vi "Read Coils.vi"(8 "error in (no error)":errorcluster, 9 "number of coils":u16, 10 "starting address":u16, 11 "Modbus master in":refnum<class "Modbus Master.lvclass">) -> (0 "error out":errorcluster, 2 "coil values":bool[](array[boolean]), 3 "Modbus master out":refnum<class "Modbus Master.lvclass">)   [LabVIEW 2020, in "Modbus Master.lvclass"]
doc: "Reads values from contiguous coils. The maximum number of coils this VI can read is 2,000."
uses:
  <vilib>/Modbus/master/Modbus Master.lvclass
  C:/builds/penguin/iak/lvdsc/trunk/20.0/lv/vi.lib/Modbus/subvis/Modbus API/Modbus API.lvclass
  <vilib>/Modbus/subvis/Modbus API/Modbus API.lvclass/Modbus API.ctl
  <vilib>/Modbus/master/Modbus Master.lvclass/Modbus Master.ctl
  <vilib>/Modbus/subvis/Protocol/Interfaces/Network Master/Network Master.lvclass
  C:/builds/penguin/iak/lvdsc/trunk/20.0/lv/vi.lib/Modbus/subvis/Protocol/Interfaces/Network Protocol/Network Protocol.lvclass
  <vilib>/Modbus/subvis/Transmission Data Unit (ADU)/Transmission Data Unit/Transmission Data Unit.lvclass
  <vilib>/Modbus/subvis/Modbus API/Modbus API.lvclass
  <vilib>/Modbus/subvis/Data and Functions/Master Function Definition/Master Function Definition.lvlib
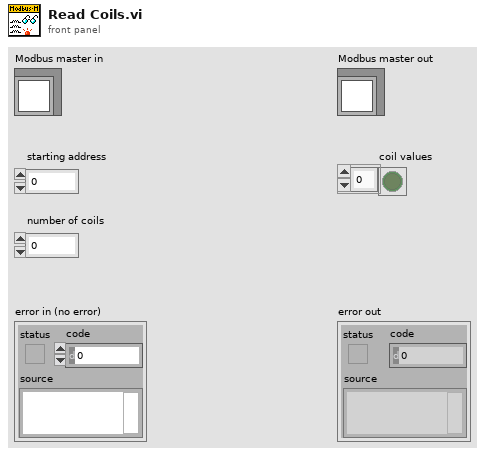
[diagram p1: front panel]
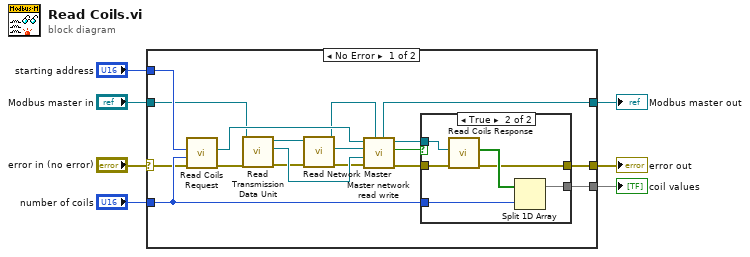
[diagram p0: block diagram]
diagram:
  n1 = case shown="No Error" "error in (no error)" {
    selector: "error in (no error)" -> [w8 w34]
    tunnel: [w19 w34] -> w5
    tunnel: [w16 w33] -> w6
    tunnel: "Modbus master in" -> [w9 w33]
    tunnel: "starting address" -> [w25 _]
    tunnel: "number of coils" -> [w24 _]
    tunnel: [w23 _] -> w4
    frame No Error {
      n2 = call <vilib>:"Read Coils Request.vi"("error in (no error)"=w8, "number of coils"=w24, "starting address"=w25) -> ("error out"=w11:errorcluster, "Modbus data unit out"=w22:refnum<class "Modbus Data Unit (PDU).lvclass">)  [unwired: 7 in]
      n3 = call <vilib>:"Read Transmission Data Unit.vi"("error in (no error)"=w11, "Modbus instance in"=w9) -> ("error out"=w14:errorcluster, "transmission data unit"=w18:refnum<class "Transmission Data Unit.lvclass">, "Modbus instance out"=w13:refnum<class "Modbus Master.lvclass">)  [unwired: 7 in]
      n4 = call <vilib>:"Read Network Master.vi"("error in (no error)"=w14, "Modbus master in"=w13) -> ("error out"=w15:errorcluster, "network master"=w17:refnum<class "Network Master.lvclass">, "Modbus master out"=w12:refnum<class "Modbus Master.lvclass">)  [unwired: 7 in]
      n5 = call <vilib>:"Master network read write.vi"("Modbus master in"=w12, "error in (no error)"=w15, "transmission data unit in"=w18, "network master in"=w17, "Modbus data unit in"=w22) -> ("error out"=w20:errorcluster, "PDU valid?"=w10:bool, "Modbus data unit out"=w21:refnum<class "Modbus Data Unit (PDU).lvclass">, "Modbus master out"=w16:refnum<class "Modbus Master.lvclass">)  [unwired: 3 in]
      n6 = case shown="True" w10 {
        tunnel: w24 -> [_ w32]
        tunnel: [_ w31] -> w23
        tunnel: w21 -> [_ w29]
        tunnel: w20 -> [w26 w28]
        tunnel: [w26 w27] -> w19
        frame False {
        }
        frame True {
          n7 = call <vilib>:"Read Coils Response.vi"("error in (no error)"=w28, "Modbus data unit in"=w29) -> ("error out"=w27:errorcluster, "data"=w30:bool[])  [unwired: 8 in]
          n8 = Split 1D Array(array=w30, index=w32) -> (first subarray=w31:bool[])  [unwired: 1 out]
        }
      }
    }
    frame Error {
    }
  }
  "error out" <- w5
  "Modbus master out" <- w6
  "coil values" <- w4
